vi "WriteFileHeader.vi"(0 "Path":path, 1 "Delimiter Character":string) -> (2 "Path Out":path)   [LabVIEW 2010]
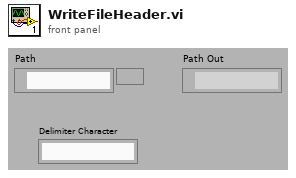
[diagram p1: front panel]
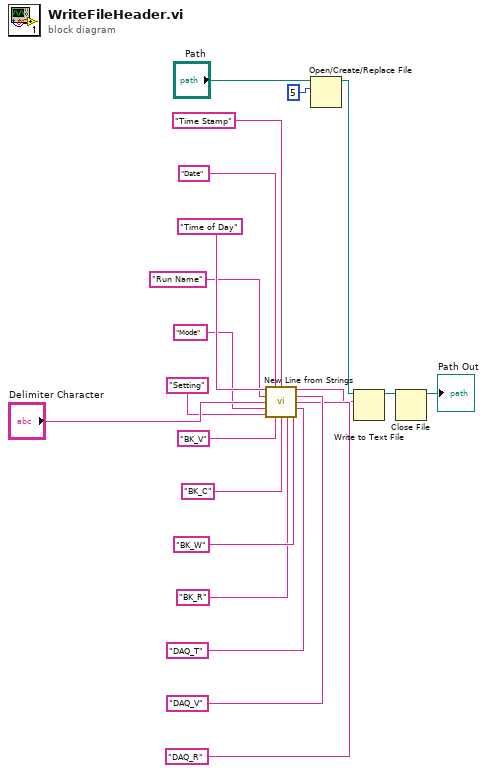
[diagram p0: block diagram]
diagram:
  n1 = call "New Line from Strings.vi"("Time"="Time of Day", "Date"="Date", "Time Stamp"="Time Stamp", "RunName"="Run Name", "DAQ Potential (milliVolts)"="DAQ_V", "Delimiter Character"="Delimiter Character", "DAQ Resistance (Ohms)"="DAQ_R", "Mode"="Mode", "DAQ Temperature (deg Celsius)"="DAQ_T", "Setting"="Setting", "BK V"="BK_V", "BK C"="BK_C", "BK R"="BK_R", "BK W"="BK_W") -> ("Line Produced"=w3:string)  [unwired: 1 in]
  n2 = Open/Create/Replace File(file path (use dialog)="Path", operation (0:open)=5) -> (refnum out=w17:refnum<file>)  [unwired: 4 in, 2 out]
  n3 = Write to Text File(file (use dialog)=w17, text=w3) -> (refnum out=w20:refnum<file>)  [unwired: 2 in, 2 out]
  n4 = Close File(refnum=w20) -> (path=→"Path Out":path)  [unwired: 1 in, 1 out]
